vi "TDMS Open Retry.vi"(4 "Lock File? (T)":bool=TRUE, 8 "error in (no error)":errorcluster, 10 "Operation (0:open)":T1(ring), 11 "Path":path) -> (0 "error out":errorcluster, 1 "Iterations":i32, 2 "TDMS Temp Path":path, 3 "TDMS File Ref":refnum<k34>)   [LabVIEW 2011]
uses:
  Summitek EXT/OpenG EXT/file/file.llb/File Exists - Scalar__ogtk.vi
  Summitek EXT/OpenG EXT/file/file.llb/Strip Path Extension - Path__ogtk.vi
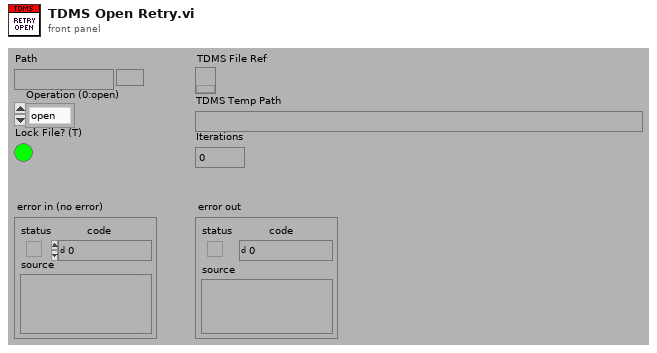
[diagram p1: front panel]
types:
  T1 = enum16{"open", "open or create", "create or replace", "create", "open (read-only)"}
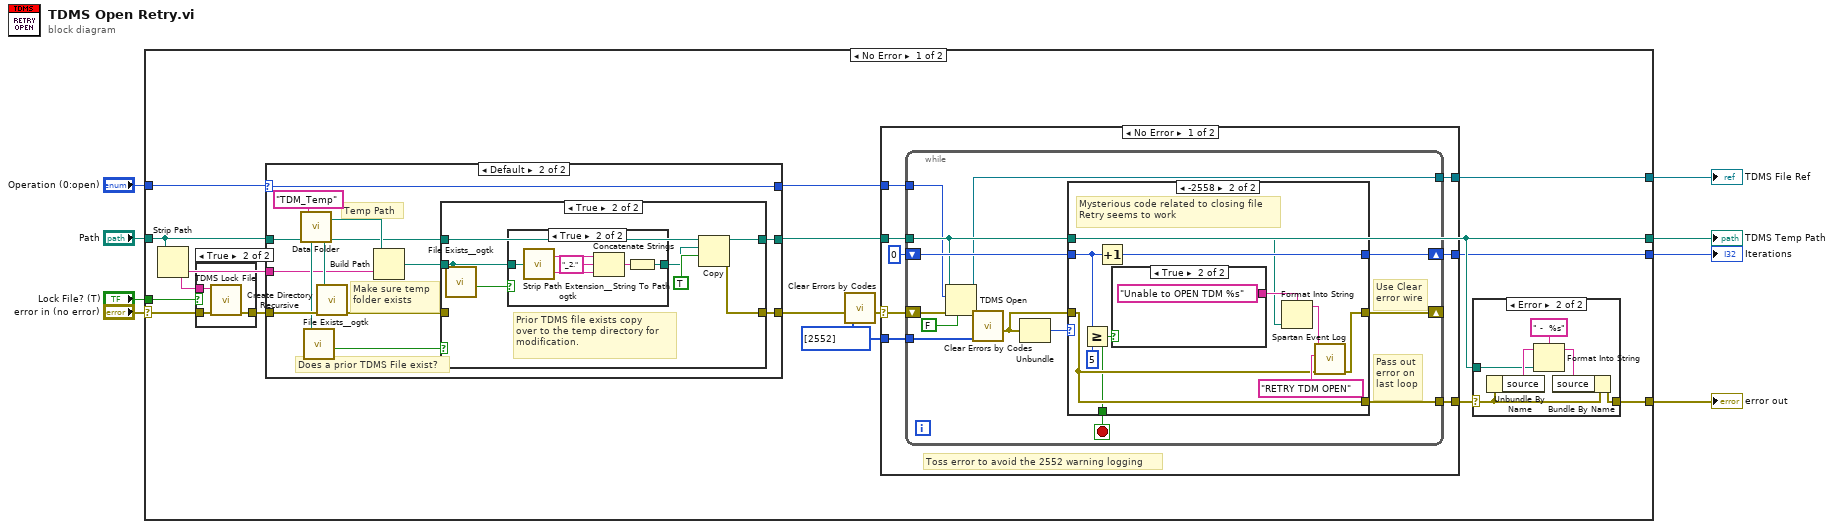
[diagram p0: block diagram]
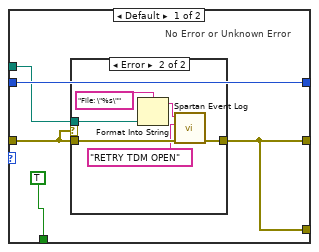
[diagram p4: hidden frame]
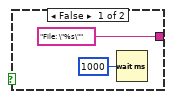
[diagram p6: hidden frame]
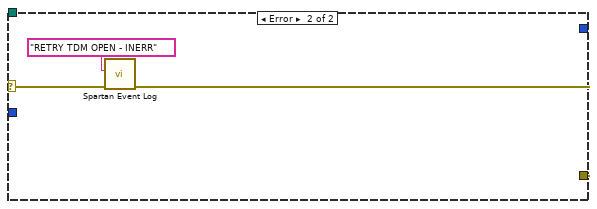
[diagram p7: hidden frame]
diagram:
  n1 = case shown="No Error" "error in (no error)" {
    selector: "error in (no error)" -> [w13 w115]
    tunnel: [w23 _] -> w2
    tunnel: "Path" -> [w12 _]
    tunnel: "Operation (0:open)" -> [w22 _]
    tunnel: [w20 _] -> w6
    tunnel: [w19 w115] -> w5
    tunnel: [w18 _] -> w4
    tunnel: "Lock File? (T)" -> [w9 _]
    frame No Error {
      w14 = i32[] [2552] ("Error Codes\nto Clear (Empty)")
      n2 = Strip Path(path=w12) -> (name=w11:string)  [unwired: 1 out]
      n3 = case shown="True" w9 {
        tunnel: w13 -> [w24 w26]
        tunnel: w11 -> [_ w27]
        tunnel: [w24 w25] -> w10
        frame False {
        }
        frame True {
          n4 = call "TDMS Lock File.vi"("error in (no error)"=w26, "Filename"=w27) -> ("error out"=w25:errorcluster)  [unwired: 9 in]
        }
      }
      n5 = case shown="Default" w22 {
        selector: w22 -> [w85 w94]
        tunnel: w10 -> [w86 w93]
        tunnel: [w87 w97] -> w20
        tunnel: w12 -> [w87 w90]
        tunnel: [w86 w95] -> w17
        tunnel: [w85 w94] -> w21
        tunnel: w11 -> [_ w88]
        frame "create or replace", "open (read-only)" {
          # "The query TDM use the \"create or replace\" mode for the files. \nThey aren't in the search area.\nRead only operations shouldn't be affected either"
        }
        frame Default {
          # "Does a prior TDMS File exist?"
          # "Make sure temp\nfolder exists"
          # "Temp Path"
          n6 = call "Data Folder.vi"("Relative Path (\"\" - Folder)"="TDM_Temp" ("Relative Path (\"\" - Folder)")) -> ("Data Folder"=w92:path)  [unwired: 2 in]
          n7 = call-poly "File Exists__ogtk.vi"("file path"=w90) -> ("exists"=w89:bool)  [unwired: 6 in, 1 out]
          n8 = call <vilib>:"Create Directory Recursive.vi"("error in (no error)"=w93, "directory"=w92) -> ("error out"=w91:errorcluster)  [unwired: 1 in, 4 out]
          n9 = Build Path(base path=w92, name or relative path=w88) -> (appended path=w96:path)
          n10 = case shown="True" w89 {
            tunnel: [w99 w107] -> w97
            tunnel: w90 -> [_ w106]
            tunnel: w96 -> [w99 w104]
            tunnel: w91 -> [w100 _]
            tunnel: [w100 w105] -> w95
            frame False {
              # "Prior TDMS Does not exist don't need\nto copy to temp directory"
            }
            frame True {
              # "Prior TDMS file exists copy \nover to the temp directory for \nmodification."
              n11 = call-poly "File Exists__ogtk.vi"("file path"=w104) -> ("exists"=w103:bool)  [unwired: 6 in, 1 out]
              n12 = case shown="True" w103 {
                tunnel: w104 -> [w108 w109]
                tunnel: [w108 w110] -> w101
                frame False {
                }
                frame True {
                  n13 = call-poly "Strip Path Extension__ogtk.vi"("path"=w109) -> ("root"=w112:string, "extension"=w111:string)
                  n14 = Concatenate Strings(w112, "_2." ("string"), w111) -> (w114:string)
                  n15 = String To Path(string=w114) -> (path=w110:path)
                }
              }
              n16 = Copy(9:TRUE ("overwrite (F)"), 10:w101, 11:w106) -> (0:w105:errorcluster, 3:w107:path)  [unwired: 1 in, 2 out]
            }
          }
        }
      }
      n17 = call "Clear Errors by Codes.vi"("Error Codes\nto Clear (Empty)"=w14, "error in (no error)"=w17) -> ("error out"=w15:errorcluster)  [unwired: 5 out]
      n18 = case shown="No Error" w15 {
        selector: w15 -> [w36 w82]
        tunnel: w20 -> [w42 _]
        tunnel: [w41 _] -> w23
        tunnel: [w40 w84] -> w16
        tunnel: w21 -> [w37 _]
        tunnel: [w38 _] -> w18
        tunnel: w14 -> [w35 _]
        frame No Error {
          # "Toss error to avoid the 2552 warning logging"
          n19 = while {
            shift-right: [w51] -> _
            shift-left: w36 -> [w49]
            shift-right: [w54] -> w38
            shift-left: 0 -> [w55]
            tunnel: w42 -> [w50]
            tunnel: [w53] -> w41
            tunnel: [w52] -> w40
            tunnel: w37 -> [w48]
            tunnel: w35 -> [w44]
            stop <- w56 stop-if-true
            # "Pass out\nerror on \nlast loop"
            # "Use Clear\nerror wire"
            n20 = TDMS Open(6:FALSE ("disable buffering (T)"), 8:w49, 10:w48, 11:w50) -> (0:w47:errorcluster, 3:w53:refnum<k34>)  [unwired: 2 in]
            n21 = call "Clear Errors by Codes.vi"("Error Codes\nto Clear (Empty)"=w44, "error in (no error)"=w47) -> ("error out"=w46:errorcluster)  [unwired: 5 out]
            n22 = Unbundle(w46) -> ("code"=w45:i32)  [unwired: 2 out]
            n23 = case shown="-2558" w45 {
              tunnel: [TRUE ("T button?") w70] -> w56
              tunnel: w46 -> [w57 w74]
              tunnel: w55 -> [w60 w76]
              tunnel: [w60 w77] -> w54
              tunnel: [w59 w74] -> w52
              tunnel: [w59 w73] -> w51
              tunnel: w50 -> [w58 w69]
              frame Default {
                # "No Error or Unknown Error"
                n24 = case shown="Error" w57 {
                  tunnel: w57 -> [w62 w68]
                  tunnel: [w62 w67] -> w59
                  tunnel: w58 -> [_ w64]
                  frame No Error {
                  }
                  frame Error {
                    n25 = Format Into String(format string="File: \"%s\"" ("message (\"\")"), w64) -> (resulting string=w65:string)  [unwired: 2 in, 1 out]
                    n26 = call "Spartan Event Log.vi"("error in (no error)"=w68, "module (\"\")"="RETRY TDM OPEN", "message (\"\")"=w65) -> ("error out"=w67:errorcluster)  [unwired: 5 in]
                  }
                }
              }
              frame -2558 {
                # "Mysterious code related to closing file\nRetry seems to work"
                n27 = Greater Or Equal?(x=w76, y=5) -> (x >= y?=w70:bool)
                n28 = Increment(x=w76) -> (x+1=w77:i32)
                n29 = case shown="True" w70 {
                  tunnel: ["File: \"%s\"" ("message (\"\")") "Unable to OPEN TDM %s" ("message (\"\")")] -> w71
                  frame False {
                    n30 = Wait (ms)(milliseconds to wait=u32 1000) -> ()  [unwired: 1 out]
                  }
                  frame True {
                  }
                }
                n31 = Format Into String(format string=w71, w69) -> (resulting string=w72:string)  [unwired: 2 in, 1 out]
                n32 = call "Spartan Event Log.vi"("error in (no error)"=w74, "module (\"\")"="RETRY TDM OPEN", "message (\"\")"=w72) -> ("error out"=w73:errorcluster)  [unwired: 5 in]
              }
            }
          }
        }
        frame Error {
          n33 = call "Spartan Event Log.vi"("error in (no error)"=w82, "module (\"\")"="RETRY TDM OPEN - INERR" ("module (\"\")")) -> ("error out"=w84:errorcluster)  [unwired: 6 in]
        }
      }
      n34 = case shown="Error" w16 {
        selector: w16 -> [w28 w31]
        tunnel: w20 -> [_ w32]
        tunnel: [w28 w29] -> w19
        frame No Error {
        }
        frame Error {
          n35 = Unbundle By Name(w31) -> ("source"=w33:string)
          n36 = Format Into String(format string=" -  %s", initial string=w33, w32) -> (resulting string=w30:string)  [unwired: 1 in, 1 out]
          n37 = Bundle By Name(cluster=w31, "source"=w30) -> (w29:errorcluster)
        }
      }
    }
    frame Error {
    }
  }
  "TDMS File Ref" <- w2
  "error out" <- w5
  "Iterations" <- w4
  "TDMS Temp Path" <- w6
